vi "SUB_creat_DAQ_Virtual_Tasks.vi"() -> (2 "SDAOUT TASK":refnum<k21>, 3 "SCK Task":refnum<k21>)   [LabVIEW 2011]
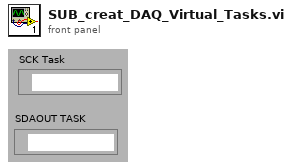
[diagram p1: front panel]
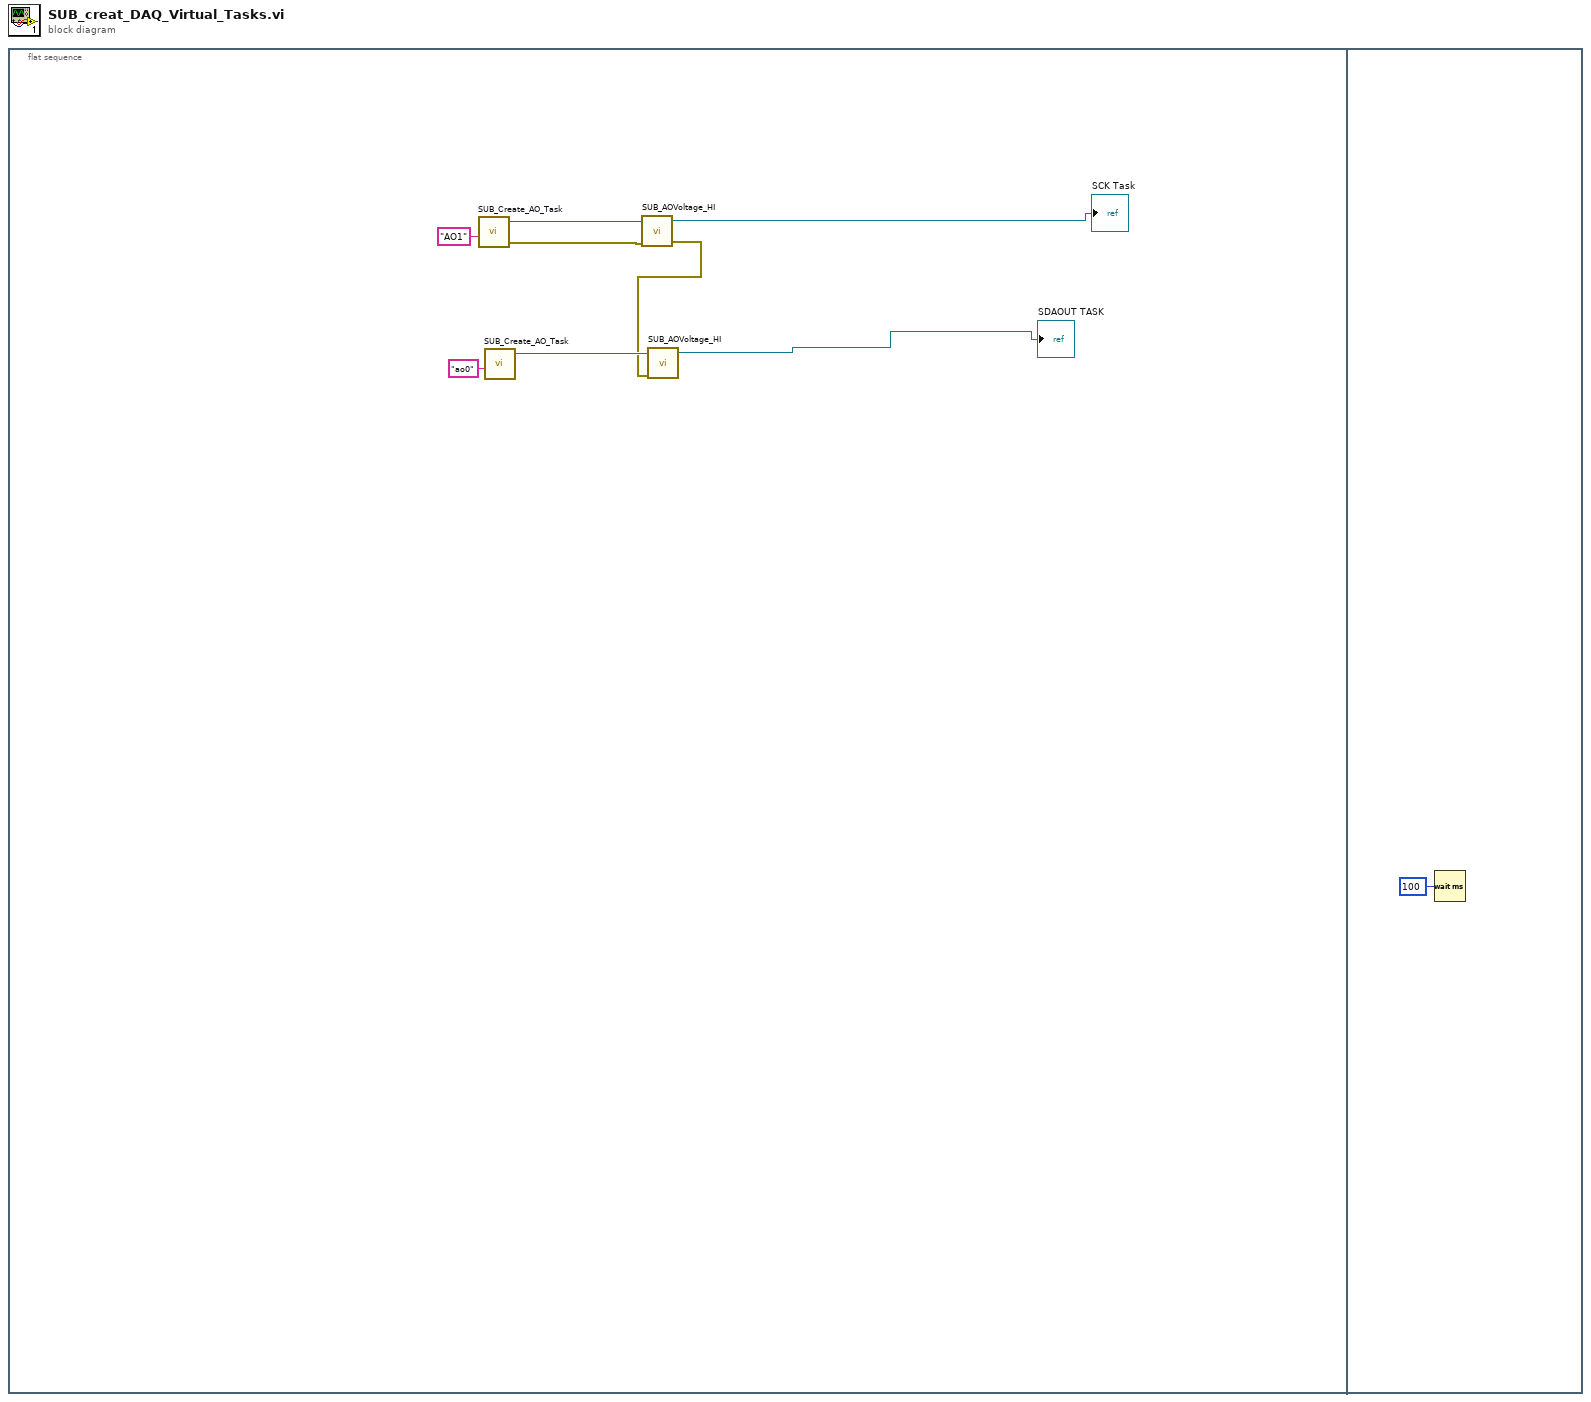
[diagram p0: block diagram]
diagram:
  n1 = flat-sequence {
    frame #0 {
      n2 = call "SUB_Create_AO_Task.vi"("Channel"="AO1") -> ("task out"=w7:refnum<k21>, "error out"=w1:errorcluster)  [unwired: 6 in]
      n3 = call "SUB_Create_AO_Task.vi"("Channel"="ao0") -> ("task out"=w4:refnum<k21>)  [unwired: 6 in, 1 out]
      n4 = call "SUB_AOVoltage_HI.vi"("task/channels in"=w7, "error in"=w1) -> ("task out"=→"SCK Task":refnum<k21>, "error out"=w2:errorcluster)  [unwired: 5 in]
      n5 = call "SUB_AOVoltage_HI.vi"("task/channels in"=w4, "error in"=w2) -> ("task out"=→"SDAOUT TASK":refnum<k21>)  [unwired: 5 in, 1 out]
    }
    frame #1 {
      n6 = Wait (ms)(milliseconds to wait=u32 100) -> ()  [unwired: 1 out]
    }
  }
